vi "Objective stage scan.vi"() -> ()   [LabVIEW 2020]
uses:
  <vilib>/DAQmx/write.llb/DAQmx Write (Analog 1D Wfm NChan NSamp).vi
  <vilib>/DAQmx/create/channels.llb/DAQmx Create Channel (AO-Voltage-Basic).vi
  <vilib>/DAQmx/configure/timing.llb/DAQmx Timing (Use Waveform).vi
  <vilib>/DAQmx/miscellaneous.llb/DAQmx Fill In Error Info.vi
  <vilib>/measure/NI_MABase.lvlib
panel:
  out "Piezo trigger (red) and Camera trigger (blue)":waveform(dbl)[](graph)=[{"t0"=timestamp(0 s since 1904-01-01), "dt"=0.001, "Y"=array[1000 elements]}, {"t0"=timestamp(0 s since 1904-01-01), "dt"=0.001, "Y"=array[1000 elements]}]
  in  "Trigger delay":dbl=180.0 format="%.2p"
  in  "Exposure time (ms)":dbl=1000.0
  out "# Samples written per channel":u32=1000
  in  "Stop":bool
  # "Find focus\nSet zero position\nMove (jog) manually by 20 slices at 2um step size (100 steps) to 40 um\nStart recording as stage moves back to focus and at -2um \nstep size (-100 steps) to -40um"
  # "Camera exposure=10ms"
  # "-2um step size, -100 steps \n500steps/sec, 10um/sec\nRed-> camera trigger\nWhite->piezo trigger"
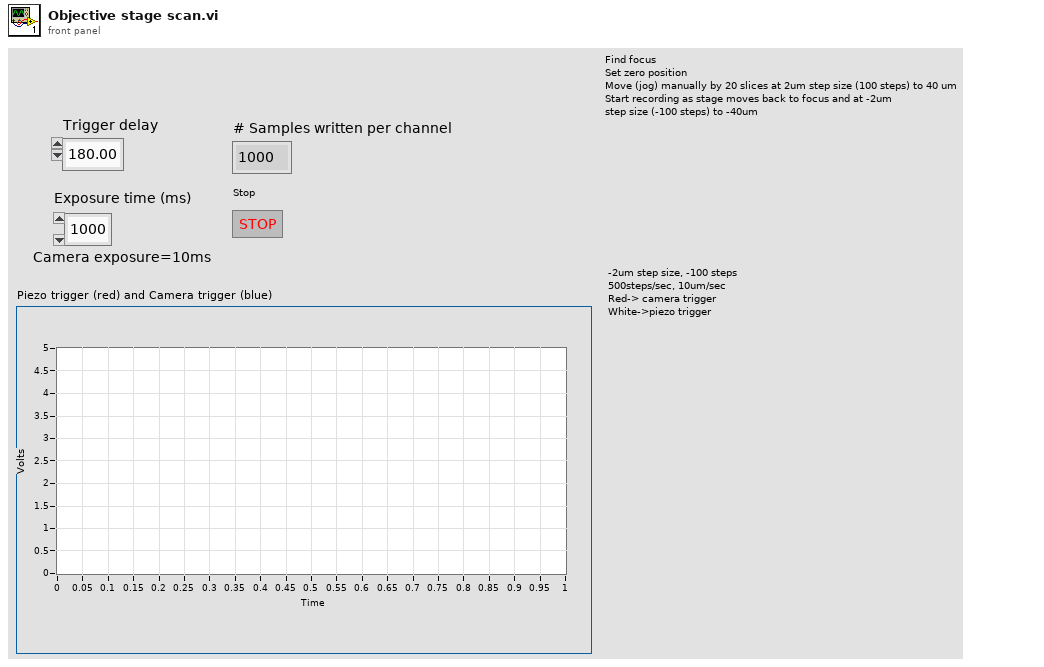
[diagram p1: front panel]
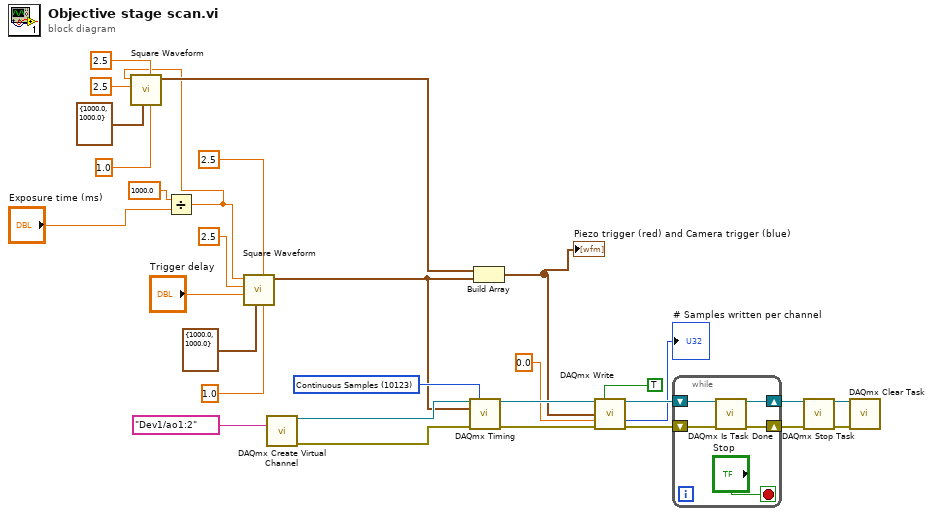
[diagram p0: block diagram]
diagram:
  w25 = 10123 items=["Finite Samples"=10178, "Continuous Samples"=10123, "Hardware Timed Single Point"=12522] ("sample mode")
  n1 = Divide(x=1000.0, y="Exposure time (ms)") -> (x/y=w2:dbl)
  n2 = call <vilib>:"Square Waveform.vi"("duty cycle (%)"=1.0, "offset"=2.5, "sampling info"=cluster{"Fs":dbl, "#s":dbl} {"Fs"=1000.0, "#s"=1000.0}, "amplitude"=2.5, "frequency"=w2) -> ("signal out"=w4:waveform(dbl))  [unwired: 5 in, 1 out]
  n3 = call <vilib>:"Square Waveform.vi"("duty cycle (%)"=1.0, "offset"=2.5, "sampling info"=cluster{"Fs":dbl, "#s":dbl} {"Fs"=1000.0, "#s"=1000.0}, "phase"="Trigger delay", "amplitude"=2.5, "frequency"=w2) -> ("signal out"=w5:waveform(dbl))  [unwired: 4 in, 1 out]
  n4 = call-poly <vilib>:"DAQmx Create Virtual Channel.vi"("physical channels"=tag "Dev1/ao1:2") -> ("task out"=w27:refnum<k21>, "error out"=w26:errorcluster)  [unwired: 13 in]
  n5 = call-poly <vilib>:"DAQmx Timing.vi"("task/channels in"=w27, "sample mode"=w25, "waveform"=w5, "error in"=w26) -> ("task out"=w22:refnum<k21>, "error out"=w21:errorcluster)  [unwired: 10 in]
  n6 = Build Array(w4, w5) -> (w1:waveform(dbl)[])
  "Piezo trigger (red) and Camera trigger (blue)" <- w1
  n7 = call-poly <vilib>:"DAQmx Write.vi"("task/channels in"=w22, "auto start"=TRUE, "data"=w1, "timeout"=0.0, "error in"=w21) -> ("task out"=w23:refnum<k21>, "number of samples written per channel"=→"# Samples written per channel":u32, "error out"=w24:errorcluster)  [unwired: 8 in]
  n8 = while {
    shift-right: [w32] -> w19
    shift-left: w23 -> [w35]
    shift-right: [w33] -> w20
    shift-left: w24 -> [w34]
    stop <- "Stop" stop-if-true
    n9 = call <vilib>:"DAQmx Is Task Done.vi"("task/channels in"=w35, "error in"=w34) -> ("task out"=w32:refnum<k21>, "error out"=w33:errorcluster)  [unwired: 11 in, 1 out]
  }
  n10 = call <vilib>:"DAQmx Stop Task.vi"("task/channels in"=w19, "error in"=w20) -> ("task out"=w28:refnum<k21>, "error out"=w29:errorcluster)  [unwired: 12 in]
  n11 = call <vilib>:"DAQmx Clear Task.vi"("task in"=w28, "error in"=w29) -> ()  [unwired: 13 in, 1 out]
